vi "FileNumber.vi"(8 "LoopIteration":i32, 11 "NumberFiles":i32) -> (1 "FileNumber":i32)   [LabVIEW 2016]
panel:
  out "x/y":dbl
  out "x-y":dbl
  out "floor(x/y)":dbl
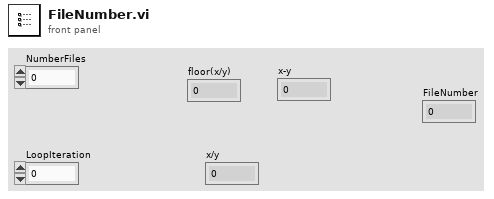
[diagram p1: front panel]
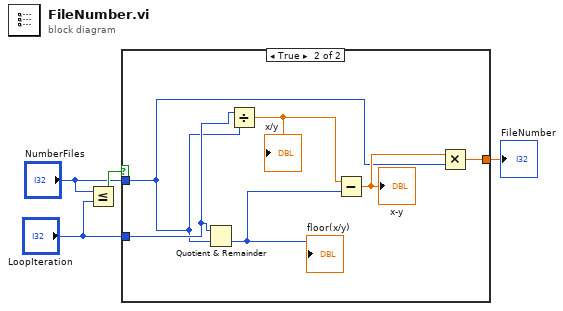
[diagram p0: block diagram]
diagram:
  n1 = Less Or Equal?(x="NumberFiles", y="LoopIteration") -> (x <= y?=w3:bool)
  n2 = case shown="True" w3 {
    tunnel: "LoopIteration" -> [w5 w7]
    tunnel: "NumberFiles" -> [_ w6]
    tunnel: [w5 w8] -> w4
    frame False {
    }
    frame True {
      n3 = Quotient & Remainder(x=w7, y=w6) -> (floor(x/y)=w10:i32)  [unwired: 1 out]
      "floor(x/y)" <- w10
      n4 = Divide(x=w7, y=w6) -> (x/y=w11:dbl)
      "x/y" <- w11
      n5 = Subtract(x=w11, y=w10) -> (x-y=w9:dbl)
      "x-y" <- w9
      n6 = Multiply(x=w9, y=w6) -> (x*y=w8:dbl)
    }
  }
  "FileNumber" <- w4
